vi "Set Configuration.vi"(8 "error in (no error)":errorcluster, 10 "configuration":T1={"name"="Channel", "units"="V", "engine data type"=enum."DBL", "string data type"=enum."DBL", "string offset"=0} {"string offset" format="%d bytes"}, 11 "Core Channel Configuration in":refnum<class "Channel Configuration.lvclass">) -> (0 "error out":errorcluster, 3 "Core Channel Configuration out":refnum<class "Channel Configuration.lvclass">)   [LabVIEW 2019, in "DSF Core.lvlib" / "Channel Configuration.lvclass"]
uses:
  Channel Configuration.lvclass
  Typedefs/Core Channel Configuration.ctl
  Typedefs/DSF Data Type.ctl
  Channel Configuration.lvclass/Channel Configuration.ctl
  DSF Core.lvlib
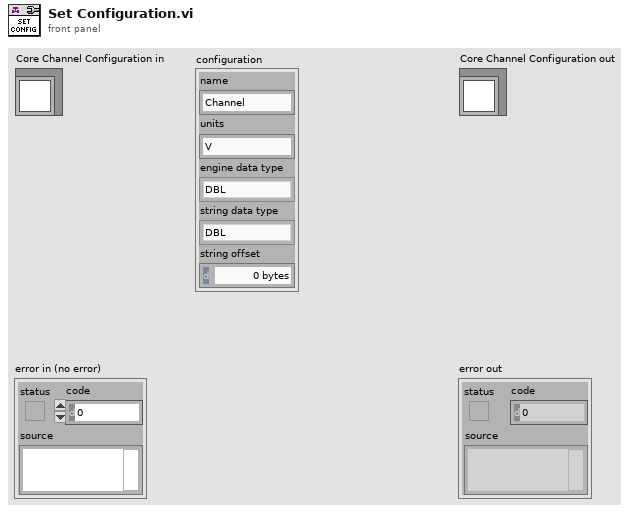
[diagram p1: front panel]
types:
  T1 = typedef "DSF Core.lvlib/Channel Configuration.lvclass/Core Channel Configuration.ctl" = cluster{"name":string, "units":string, "engine data type":T2, "string data type":T2, "string offset":u64}
  T2 = typedef "DSF Core.lvlib/DSF Data Type.ctl" = enum8{"Bool", "SGL", "DBL", "I8", "I16", "I32", "I64", "U8", "U16", "U32", "U64"}
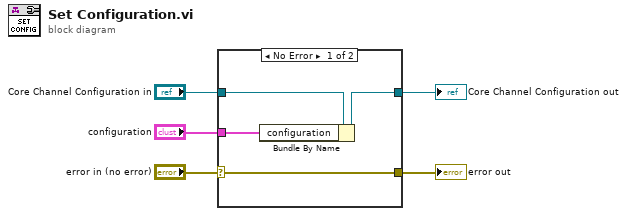
[diagram p0: block diagram]
diagram:
  n1 = case shown="No Error" "error in (no error)" {
    selector: "error in (no error)" -> [w6 w11]
    tunnel: "Core Channel Configuration in" -> [w9 w10]
    tunnel: "configuration" -> [w8 _]
    tunnel: [w7 w10] -> w3
    tunnel: [w6 w11] -> w1
    frame No Error {
      n2 = Bundle By Name(cluster=w9, "configuration"=w8) -> (w7:refnum<class "Channel Configuration.lvclass">)
    }
    frame Error {
    }
  }
  "error out" <- w1
  "Core Channel Configuration out" <- w3
